vi "Close DMM.vi"(8 "error in (no error)":errorcluster, 11 "DMM Driver in":refnum<class "DMM Driver.lvclass">) -> (0 "error out":errorcluster, 3 "DMM Driver out":refnum<class "DMM Driver.lvclass">)   [LabVIEW 2020, in "DMM Driver.lvclass"]
uses:
  DMM Driver.lvclass
  DMM Driver.lvclass/DMM Driver.ctl
  DMM/DMM.lvclass
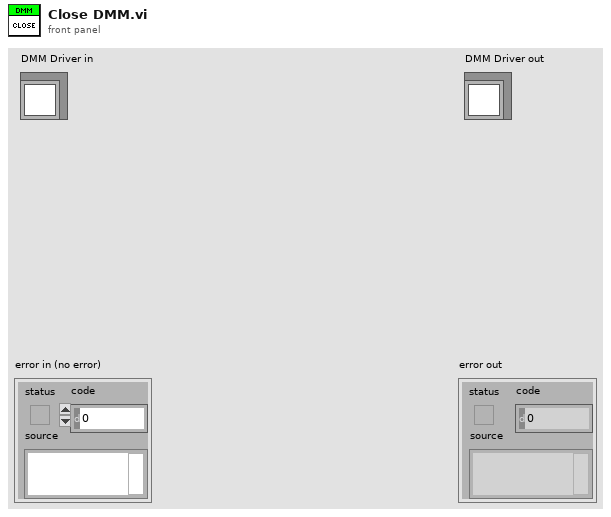
[diagram p1: front panel]
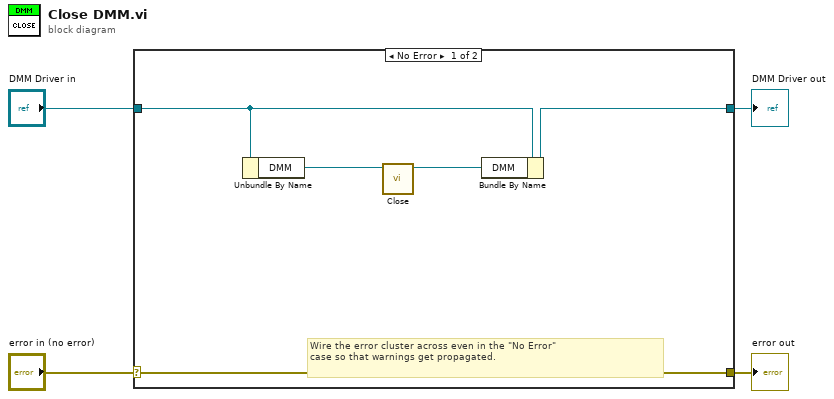
[diagram p0: block diagram]
diagram:
  n1 = case shown="No Error" "error in (no error)" {
    selector: "error in (no error)" -> [w9 w11]
    tunnel: [w9 w11] -> w3
    tunnel: [w5 w10] -> w1
    tunnel: "DMM Driver in" -> [w6 w10]
    frame No Error {
      # "Wire the error cluster across even in the \"No Error\"\ncase so that warnings get propagated."
      n2 = Unbundle By Name(w6) -> ("DMM"=w8:refnum<class "DMM.lvclass">)
      n3 = call-dynamic "Close.vi"("DMM in"=w8) -> ("DMM out"=w7:refnum<class "DMM.lvclass">)  [unwired: 9 in, 1 out]
      n4 = Bundle By Name(cluster=w6, "DMM"=w7) -> (w5:refnum<class "DMM Driver.lvclass">)
    }
    frame Error {
    }
  }
  "error out" <- w3
  "DMM Driver out" <- w1
